vi "Preference_global.vi"() -> ()   [LabVIEW 2021]
uses:
  Controls/Server_Comms.ctl
panel:
  out "Preferences for computer":path
  in  "Site Specific String (Blank if Surrey)":string
  out "MaxDailyEmails":u32=50
  in  "Send Emails?":bool
  in  "SMTP server IP address":string="Run EnFlo Hub.vi"
  in  "LabVIEW Administrators":string[](array[string])
  in  "Unblock Email":bool
  in  "HaveIMAQlibrary":bool
  in  "Log Cameras if available":bool
  in  "Project Name":string="NotSet"
  in  "User_Name":string
  in  "Rig Setup":string
  in  "Use New Collision Code":bool
  out "Traverse to Traverse Collision Detection":bool
  in  "Default Source Establishment Time (s)":dbl=20.0
  out "Application:Version Number":string
  out "Operating System:Version Number":string
  out "Operating System:Name":string
  in  "% Error From Previous Calib":dbl=0.5 format="%.1f"
  in  "Tunnel Speed Control":bool
  in  "Abs Press (mbar)":string="Run EnFlo Hub.vi"
  in  "Temperature":string="Run EnFlo Hub.vi"
  in  "Server port number":u32=3363
  in  "Server address":string="Please Run EnFlo Hub.vi"
  in  "Server Comms":T1
  # "Deg C"
  # "Warning Levels for Autocalibration Changes"
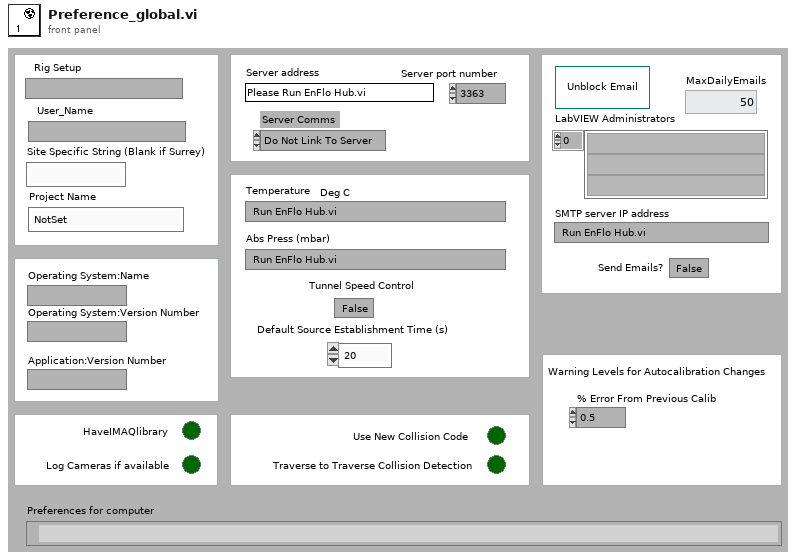
[diagram p1: front panel]
types:
  T1 = typedef "Server_Comms.ctl" = enum16{"Do Not Link To Server", "Server Link Healthy"}
diagram:
